vi "DAQNaviGet_Buffered_CI_ChannelCount.vi"(8 "error in (no error)":errorcluster, 11 "task in":i32) -> (0 "error out":errorcluster, 2 "channelCount":i32, 3 "task out":i32)   [LabVIEW 2020]
uses:
  DAQNavi_LV.dll
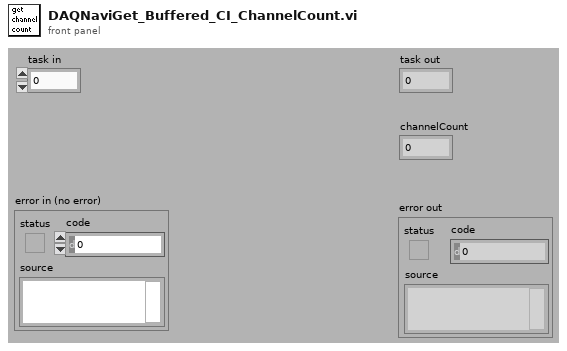
[diagram p1: front panel]
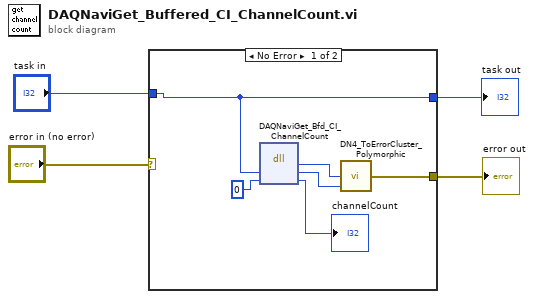
[diagram p0: block diagram]
diagram:
  n1 = case shown="No Error" "error in (no error)" {
    selector: "error in (no error)" -> [_ w11]
    tunnel: "task in" -> [w10 w12]
    tunnel: [w10 w12] -> w2
    tunnel: [w6 w11] -> w1
    frame No Error {
      n2 = dll-call lib="DAQNavi_LV.dll" fn="DAQNaviGet_Bfd_CI_ChannelCount"("taskID"=w10, "channelCount"=0) -> ("return type"=w7:i32, "taskID"=w5:i32, "channelCount"=→"channelCount":i32)  [unwired: 3 in, 2 out]
      n3 = call "DN4_ToErrorCluster_Polymorphic.vi"("task id"=w5, "error code"=w7) -> ("error out"=w6:errorcluster)  [unwired: 3 out]
    }
    frame Error {
    }
  }
  "task out" <- w2
  "error out" <- w1
